vi "Send Command.vi"(8 "error in":errorcluster, 9 "Data":u16[](array[numeric]), 10 "Command":u16 format="%.0x", 11 "FPGA VI Reference In":T1) -> (0 "error out":errorcluster, 3 "FPGA VI Reference Out":T1)   [LabVIEW 2019]
uses:
  TypeDefs/FPGA Reference.ctl
  TypeDefs/Type of message.ctl
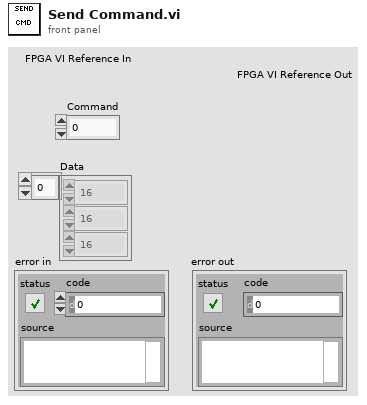
[diagram p1: front panel]
types:
  T1 = typedef "FPGA Reference.ctl" = refnum<k20>
  T2 = typedef "Type of message.ctl" = enum16{"CMD", "DATA"}
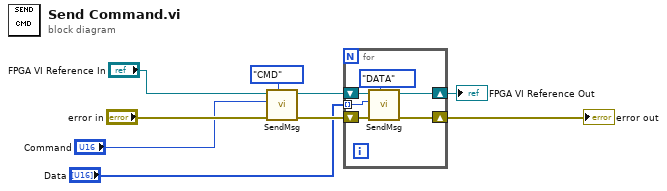
[diagram p0: block diagram]
diagram:
  n1 = call "SendMsg.vi"("MsgType"=Type_of_message."CMD", "error in"="error in", "Payload"="Command", "FPGA VI Reference Out 2"="FPGA VI Reference In") -> ("error out"=w6:errorcluster, "FPGA VI Reference Out"=w5:T1)  [unwired: 5 in, 1 out]
  n2 = for {
    shift-right: [w13] -> w4
    shift-left: w6 -> [w15]
    shift-right: [w12] -> w1
    shift-left: w5 -> [w14]
    tunnel: "Data" -> [w10] mode=indexing
    n3 = call "SendMsg.vi"("MsgType"=Type_of_message."DATA", "error in"=w15, "Payload"=w10, "FPGA VI Reference Out 2"=w14) -> ("error out"=w13:errorcluster, "FPGA VI Reference Out"=w12:T1)  [unwired: 5 in, 1 out]
  }
  "error out" <- w4
  "FPGA VI Reference Out" <- w1
